vi "StringToCSG.vi"(0 "String":string, 7 "Offset":i32 caption="Offset (0)", 11 "Error in":errorcluster caption="Error in (no error)") -> (4 "Complex number":csg, 15 "Error out":errorcluster)   [LabVIEW 2017, in "GPString.lvlib"]
doc: "Converts <B>String</B> to <B>Complex number</B>, starting the conversion from the optional <B>Offset</B> in <B>String</B>.\n\n<B>String formatting</B>\n- Both period (.) and comma (,) are supported as radix point in <B>String</B>.\n- Both parantheses-form \"(7.8,-9)\" and imaginary unit-form \"-4+3.1i\" are allowed.\n- For parantheses-form use either \";\" or \",\" (only with radix point=\".\") as re/im separator.\n- Both \"i\" and \"j\" are allowed as imaginary unit.\n- Imaginary unit may be stated as \"*i\" or simply as \"i\", but always after the imaginary number part.\n- <B>String</B> may contain numbers without imaginary part (e.g. \"-3\") and without real part (e.g. \"-2.9i\" or \"-i\").\n\nThis VI is inlined.\n\nSteen Schmidt\nGPower\n15/6 2016"
uses:
  GPString.lvlib
panel:
  # "Copyright © 2015\nGPower\nSee enclosed license file for terms and conditions"
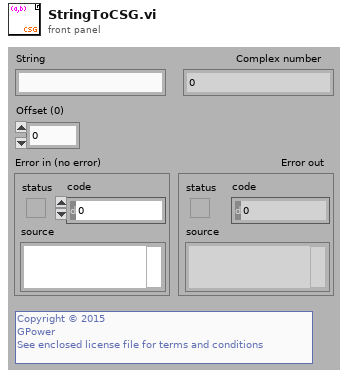
[diagram p1: front panel]
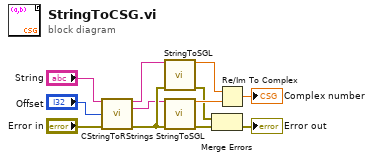
[diagram p0: block diagram]
diagram:
  n1 = call "CStringToRStrings.vi"("Complex string"="String", "Offset"="Offset", "Error in"="Error in") -> ("Real string"=w8:string, "Imaginary string"=w9:string, "Error out"=w10:errorcluster)  [unwired: 10 in]
  n2 = call "StringToSGL.vi"("String"=w8, "Error in"=w10) -> ("Number"=w7:sgl, "Error out"=w4:errorcluster)  [unwired: 11 in, 1 out]
  n3 = call "StringToSGL.vi"("String"=w9, "Error in"=w10) -> ("Number"=w6:sgl, "Error out"=w3:errorcluster)  [unwired: 11 in, 1 out]
  n4 = Merge Errors(w4, w3) -> (→"Error out":errorcluster)
  n5 = Re/Im To Complex(1:w6, 2:w7) -> (0:→"Complex number":csg)
